vi "CRYGet Fonts.vi"() -> (3 "Fonts out":string[](array[string]))   [LabVIEW 2013]
uses:
  <vilib>/registry/registry.llb/Registry RtKey.ctl
  <vilib>/registry/registry.llb/Registry SAM.ctl
panel:
  # "Get System Font Names"
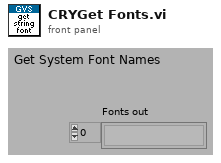
[diagram p1: front panel]
types:
  T1 = typedef "Registry SAM.ctl" = enum32{"KEY_QUERY_VALUE", "KEY_SET_VALUE", "KEY_CREATE_SUB_KEY", "KEY_ENUMERATE_SUB_KEYS", "KEY_NOTIFY", "KEY_CREATE_LINK", "KEY_READ", "KEY_WRITE", "KEY_ALL_ACCESS", "KEY_READ | KEY_WRITE"}
  T2 = typedef "Registry RtKey.ctl" = enum32{"HKEY_CLASSES_ROOT", "HKEY_CURRENT_USER", "HKEY_LOCAL_MACHINE", "HKEY_USERS", "HKEY_PERFORMANCE_DATA", "HKEY_CURRENT_CONFIG", "HKEY_DYN_DATA"}
  T3 = typedef "Registry refnum.ctl" = refnum<k1>
  T4 = cluster{"numValues":i32, "maxValueNameLen":i32, "maxValueDataLen":i32}
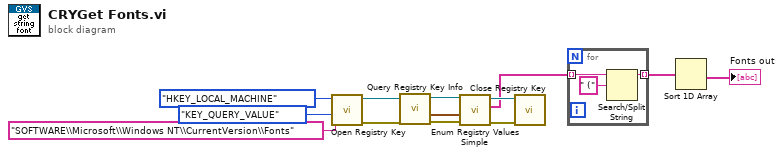
[diagram p0: block diagram]
diagram:
  n1 = call <vilib>:"Open Registry Key.vi"("security access mask (KEY_READ | KEY_WRITE)"=Registry_SAM."KEY_QUERY_VALUE", "subkey"="SOFTWARE\\Microsoft\\Windows NT\\CurrentVersion\\Fonts", "root key (HKEY_LOCAL_MACHINE)"=Registry_RtKey."HKEY_LOCAL_MACHINE") -> ("error out"=w6:errorcluster, "refnum out"=w8:T3)  [unwired: 1 in, 6 out]
  n2 = call <vilib>:"Query Registry Key Info.vi"("error in (no error)"=w6, "refnum"=w8) -> ("error out"=w5:errorcluster, "value info"=w10:T4, "refnum out"=w9:T3)  [unwired: 7 out]
  n3 = call <vilib>:"Enum Registry Values Simple.vi"("error in (no error)"=w5, "value info"=w10, "refnum"=w9) -> ("error out"=w4:errorcluster, "values"=w2:string[], "refnum out"=w11:T3)  [unwired: 1 in, 5 out]
  n4 = call <vilib>:"Close Registry Key.vi"("error in (no error)"=w4, "refnum"=w11) -> ()  [unwired: 6 out]
  n5 = for {
    tunnel: w2 -> [w15] mode=indexing
    tunnel: [w14] -> w1 mode=indexing
    n6 = Search/Split String(string=w15, search string/char (-)=" (") -> (substring before match=w14:string)  [unwired: 3 out]
  }
  n7 = Sort 1D Array(array=w1) -> (sorted array=→"Fonts out":string[])
